vi "CRYImp wiz header to curve names.vi"(9 "x-y settings array":T1=[{"x col"=0, "x data type"=0, "x axis type"=0, "x prefix"="", "x unit"="", "x db ref"=0.0, "y col"=0, "Name:"="", "phase incl"=FALSE, "ym data type"=0, "ym axis type"=0, "ym prefix"="", "ym unit"="", "ym db ref"=0.0, "yp data type"=0, "yp axis type"=0, "yp prefix"="", "yp unit"="", "yp db ref"=0.0}] {"yp db ref" format="%.2f"; "ym db ref" format="%.2f"; "x db ref" format="%.2f"}, 10 "Main info cluster":T2, 11 "Data file table":string[][](array[string])) -> (1 "x-y settings array out":T1 {"yp db ref" format="%.2f"; "ym db ref" format="%.2f"; "x db ref" format="%.2f"})   [LabVIEW 2013]
uses:
  Control/CRYImp wiz main info.ctl
  Control/CRYx-y settings array.ctl
  CRYImp wiz global.vi
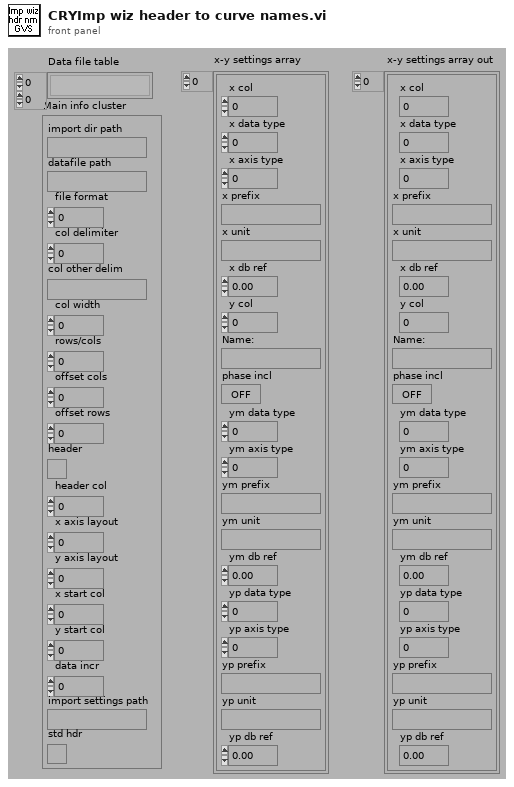
[diagram p1: front panel]
types:
  T1 = typedef "CRYx-y settings array.ctl" = cluster{"x col":i32, "x data type":u16, "x axis type":u16, "x prefix":string, "x unit":string, "x db ref":dbl, "y col":i32, "Name:":string, "phase incl":bool, "ym data type":u16, "ym axis type":u16, "ym prefix":string, "ym unit":string, "ym db ref":dbl, "yp data type":u16, "yp axis type":u16, "yp prefix":string, "yp unit":string, "yp db ref":dbl}[]
  T2 = typedef "CRYImp wiz main info.ctl" = cluster{"import dir path":path, "datafile path":path, "file format":i32, "col delimiter":i32, "col other delim":string, "col width":i32, "rows/cols":i32, "offset cols":i32, "offset rows":i32, "header":bool, "header col":i32, "x axis layout":i32, "y axis layout":i32, "x start col":i32, "y start col":i32, "data incr":i32, "import settings path":path, "std hdr":bool}
  T3 = cluster{"x col":i32, "x data type":u16, "x axis type":u16, "x prefix":string, "x unit":string, "x db ref":dbl, "y col":i32, "Name:":string, "phase incl":bool, "ym data type":u16, "ym axis type":u16, "ym prefix":string, "ym unit":string, "ym db ref":dbl, "yp data type":u16, "yp axis type":u16, "yp prefix":string, "yp unit":string, "yp db ref":dbl}
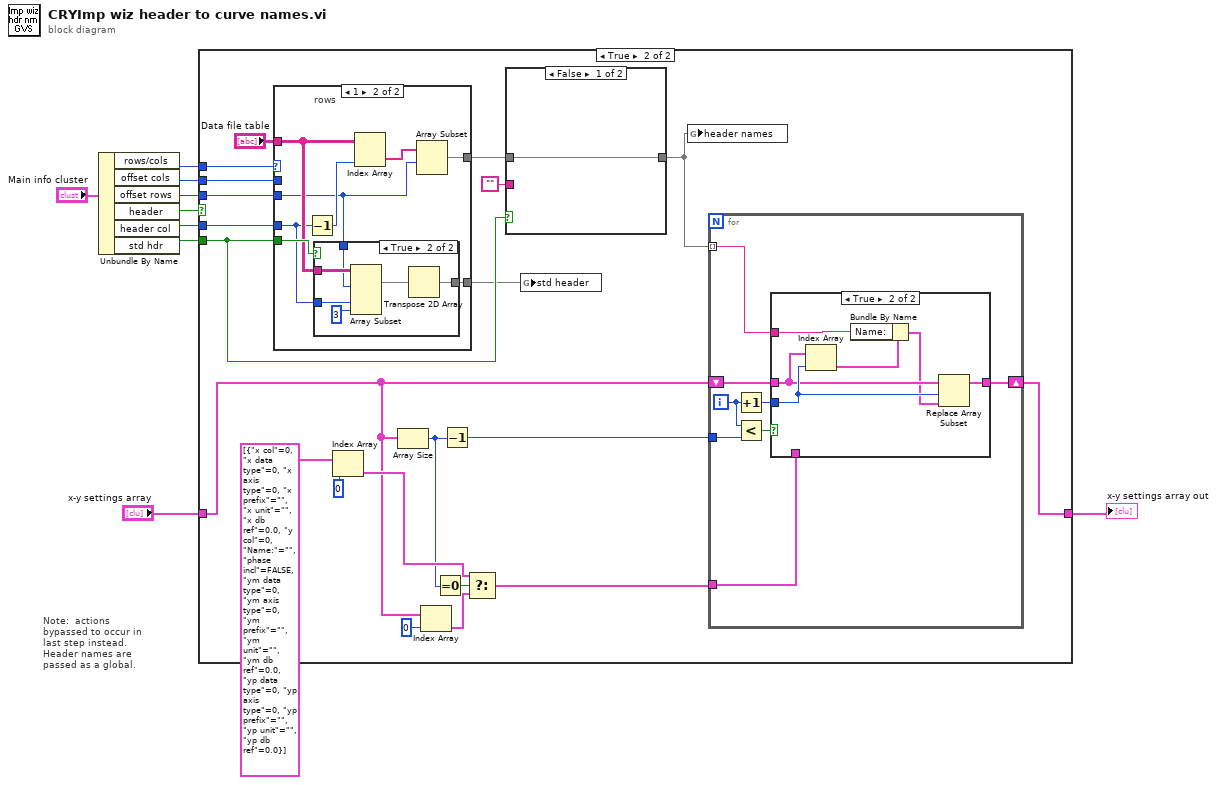
[diagram p0: block diagram]
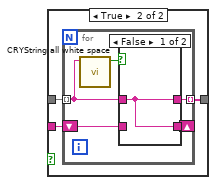
[diagram p3: hidden frame]
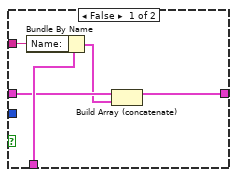
[diagram p5: hidden frame]
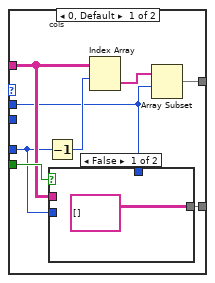
[diagram p6: hidden frame]
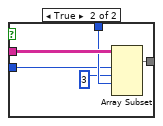
[diagram p7: hidden frame]
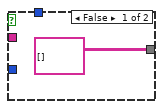
[diagram p8: hidden frame]
diagram:
  # "Note:  actions bypassed to occur in last step instead.\nHeader names are passed as a global."
  n1 = Unbundle By Name("Main info cluster") -> ("rows/cols"=w8:i32, "offset cols"=w7:i32, "offset rows"=w6:i32, "header"=w5:bool, "header col"=w4:i32, "std hdr"=w2:bool)
  n2 = case shown="True" w5 {
    tunnel: "x-y settings array" -> [w10 w19]
    tunnel: w8 -> [_ w26]
    tunnel: w7 -> [_ w25]
    tunnel: w6 -> [_ w24]
    tunnel: w4 -> [_ w23]
    tunnel: [w10 w17] -> w1
    tunnel: w2 -> [_ w13]
    frame False {
    }
    frame True {
      n3 = case shown="1" w26 {
        tunnel: w25 -> [w64 _]
        tunnel: w24 -> [_ w76]
        tunnel: w23 -> [w63 w78]
        tunnel: "Data file table" -> [w65 w79]
        tunnel: [w67 w81] -> w14
        tunnel: w13 -> [w66 w80]
        tunnel: [w62 w77] -> w11
        frame 0, Default {
          # "cols"
          n4 = Decrement(x=w63) -> (x-1=w68:i32)
          n5 = case shown="False" w66 {
            tunnel: w65 -> [_ w75]
            tunnel: w64 -> [_ w74]
            tunnel: w63 -> [_ w73]
            tunnel: [string[][] [] w71] -> w62
            frame False {
            }
            frame True {
              n6 = Array Subset(array=w75, index (row)=w73, length (row)=3 ("Array Length"), index (col)=w74) -> (w71:string[][])  [unwired: 1 in]
            }
          }
          n7 = Index Array(array=w65, index (row)=w68) -> (element=w69:string[])  [unwired: 1 in]
          n8 = Array Subset(array=w69, index=w64) -> (w67:string[])  [unwired: 1 in]
        }
        frame 1 {
          # "rows"
          n9 = Decrement(x=w78) -> (x-1=w82:i32)
          n10 = case shown="True" w80 {
            tunnel: w79 -> [_ w90]
            tunnel: w78 -> [_ w89]
            tunnel: w76 -> [_ w87]
            tunnel: [string[][] [] w85] -> w77
            frame False {
            }
            frame True {
              n11 = Array Subset(array=w90, index (row)=w87, index (col)=w89, length (col)=3 ("Array Length")) -> (w86:string[][])  [unwired: 1 in]
              n12 = Transpose 2D Array(2D array=w86) -> (transposed array=w85:string[][])
            }
          }
          n13 = Index Array(array=w79, index (col)=w82) -> (element=w83:string[])  [unwired: 1 in]
          n14 = Array Subset(array=w83, index=w76) -> (w81:string[])  [unwired: 1 in]
        }
      }
      n15 = Index Array(array=T1 [{"x col"=0, "x data type"=0, "x axis type"=0, "x prefix"="", "x unit"="", "x db ref"=0.0, "y col"=0, "Name:"="", "phase incl"=FALSE, "ym data type"=0, "ym axis type"=0, "ym prefix"="", "ym unit"="", "ym db ref"=0.0, "yp data type"=0, "yp axis type"=0, "yp prefix"="", "yp unit"="", "yp db ref"=0.0}] ("x-y settings array"), index=0 ("Dimension Size")) -> (element=w20:T3)
      n16 = Array Size(array=w19) -> (size(s)=w18:i32)
      n17 = Index Array(array=w19, index=0 ("Index")) -> (element=w27:T3)
      n18 = Equal To 0?(x=w18) -> (x = 0?=w29:bool)
      n19 = Decrement(x=w18) -> (x-1=w16:i32)
      n20 = Select(t=w20, s=w29, f=w27) -> (s? t:f=w21:T3)
      n21 = case shown="False" w13 {
        tunnel: "" -> [_ w35]
        tunnel: w14 -> [w32 w34]
        tunnel: [w32 w33] -> w12
        frame False {
        }
        frame True {
          n22 = for {
            shift-right: [w37] -> _
            shift-left: w35 -> [w36]
            tunnel: w34 -> [w39] mode=indexing
            tunnel: [w38] -> w33 mode=indexing
            n23 = call "CRYString all white space.vi"("String"=w39) -> ("Nothing but white space?"=w40:bool)  [unwired: 10 in]
            n24 = case shown="False" w40 {
              tunnel: [w41 w42] -> w38
              tunnel: w39 -> [w41 _]
              tunnel: [w41 w42] -> w37
              tunnel: w36 -> [_ w42]
              frame False {
              }
              frame True {
              }
            }
          }
        }
      }
      n25 = global write "CRYImp wiz global.vi" "std header"(w11) -> ()
      n26 = global write "CRYImp wiz global.vi" "header names"(w12) -> ()
      n27 = for {
        tunnel: w12 -> [w45] mode=indexing
        tunnel: w21 -> [w43]
        shift-right: [w44] -> w17
        shift-left: w19 -> [w48]
        tunnel: w16 -> [w50]
        i -> [w47]
        n28 = Increment(x=w47) -> (x+1=w46:i32)
        n29 = Less?(x=w47, y=w50) -> (x < y?=w49:bool)
        n30 = case shown="True" w49 {
          tunnel: w48 -> [w53 w60]
          tunnel: w46 -> [_ w61]
          tunnel: w45 -> [w55 w59]
          tunnel: [w51 w56] -> w44
          tunnel: w43 -> [w54 _]
          frame False {
            n31 = Bundle By Name(cluster=w54, "Name:"=w55) -> (w52:T3)
            n32 = Build Array (concatenate)(w53, w52) -> (w51:T1)
          }
          frame True {
            n33 = Index Array(array=w60, index=w61) -> (element=w58:T3)
            n34 = Bundle By Name(cluster=w58, "Name:"=w59) -> (w57:T3)
            n35 = Replace Array Subset(array=w60, new element=w57, index=w61) -> (w56:T1)
          }
        }
      }
    }
  }
  "x-y settings array out" <- w1
